vi "6_12_vector_matrix_multiply.vi"(1 "p":i32, 2 "n":i32, 3 "B":fxp<+/-,6,12>[](array[numeric]), 4 "A":fxp<+/-,6,12>[](array[numeric])) -> (0 "C":fxp<+/-,6,12>[](array[numeric]))   [LabVIEW 2020]
panel:
  in  "accum":fxp<+/-,6,12>
  in  "C_type":fxp<+/-,6,12>
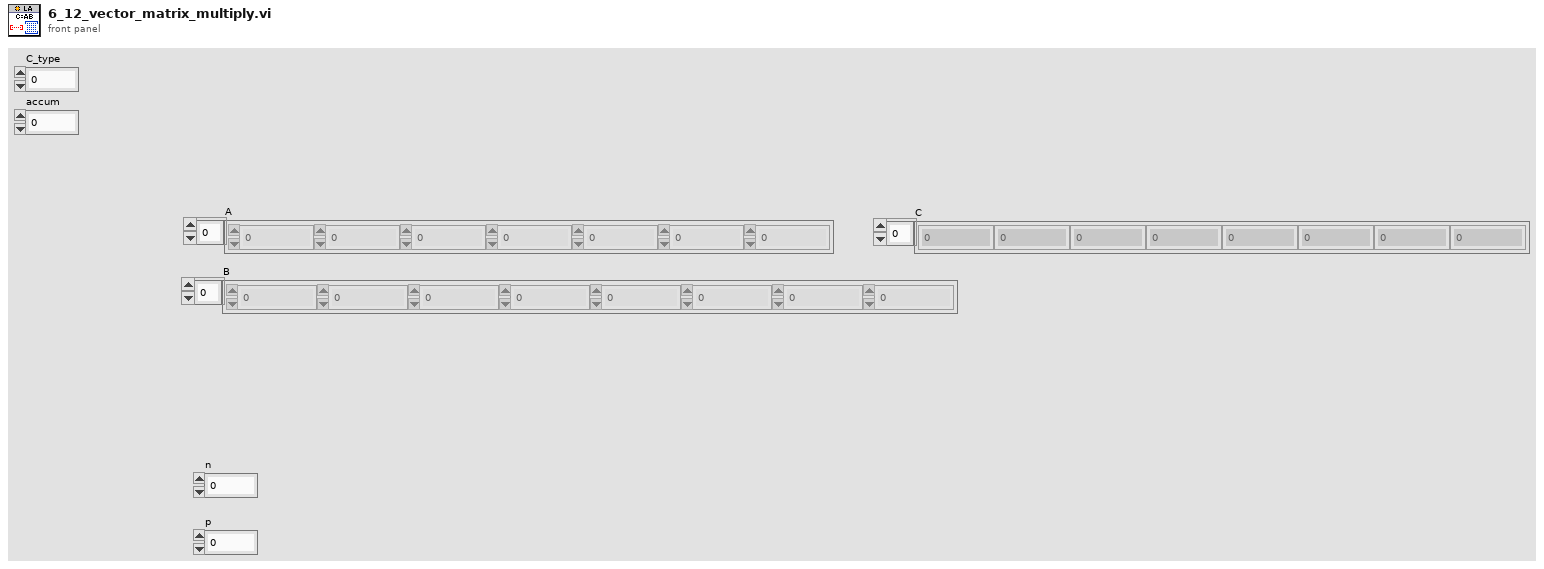
[diagram p1: front panel]
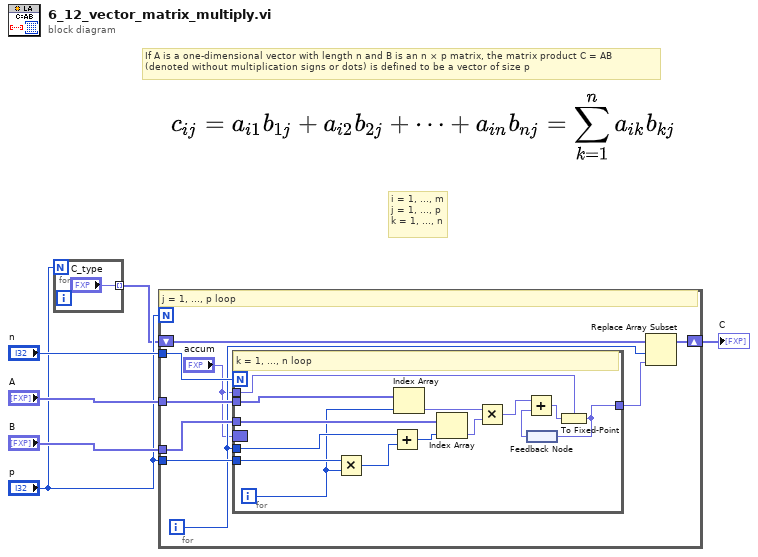
[diagram p0: block diagram]
diagram:
  # "If A is a one-dimensional vector with length n and B is an n × p matrix, the matrix product C = AB \n(denoted without multiplication signs or dots) is defined to be a vector of size p"
  # "i = 1, ..., m\nj = 1, ..., p\nk = 1, ..., n"
  n1 = for {
    N: "p" -> [_]
    tunnel: ["C_type"] -> w1 mode=indexing
  }
  n2 = for {
    N: "p" -> [_]
    tunnel: "A" -> [w16]
    tunnel: "B" -> [w15]
    tunnel: "n" -> [w11]
    tunnel: "p" -> [w10]
    shift-right: [w13] -> w4
    shift-left: w1 -> [w14]
    i -> [w9]
    # "j = 1, ..., p loop"
    n3 = for {
      N: w11 -> [_]
      tunnel: w16 -> [w30]
      tunnel: w15 -> [w29]
      tunnel: w9 -> [w24]
      tunnel: [w18] -> w12
      tunnel: w10 -> [w23]
      border: "accum" -> [_]
      tunnel: "accum" -> [w17]
      i -> [w20]
      # "k = 1, ..., n loop"
      n4 = Multiply(x=w23, y=w20) -> (x*y=w22:i32)
      n5 = Add(x=w24, y=w22) -> (x+y=w21:i32)
      n6 = Index Array(array=w30, index=w20) -> (element=w28:fxp<+/-,6,12>)
      n7 = Index Array(array=w29, index=w21) -> (element=w27:fxp<+/-,6,12>)
      n8 = Multiply(x=w28, y=w27) -> (x*y=w26:fxp<+/-,12,24>)
      n9 = feedback #1() -> (w25:fxp<+/-,6,12>)
      n10 = Add(x=w26, y=w25) -> (x+y=w19:fxp<+/-,18,24>)
      n11 = To Fixed-Point(fixed-point type=w17, number=w19) -> (fixed-point=w18:fxp<+/-,6,12>)
      n12 = feedback-in #1(w18) -> ()
    }
    n13 = Replace Array Subset(array=w14, new element=w12, index=w9) -> (w13:fxp<+/-,6,12>[])
  }
  "C" <- w4
